vi "ReadNet_ONXX.vi"(8 "error in":errorcluster, 11 "ModelPath":path) -> (0 "error out":errorcluster, 3 "NET":refnum<class "NET.lvclass">)   [LabVIEW 2020, in "OpenLvVision_OpenCv.lvlib"]
doc: "Reads a network model ONNX."
uses:
  OpenLvVision_OpenCv.lvlib
  NET/NET.lvclass
  _LvHelpers/EdvrObject/TypeDef/Edvr.ctl
  _LvHelpers/EdvrObject/EdvrObject.lvclass
  Dlls/OlvOpenCvWrapper.dll
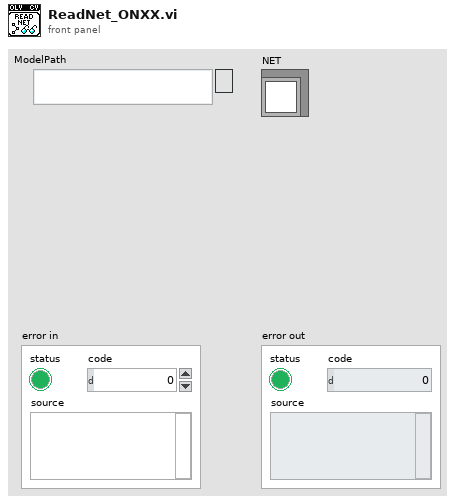
[diagram p1: front panel]
types:
  T1 = typedef "OpenLvVision_OpenCv.lvlib/EdvrObject.lvclass/Edvr.ctl" = refnum<data-value>
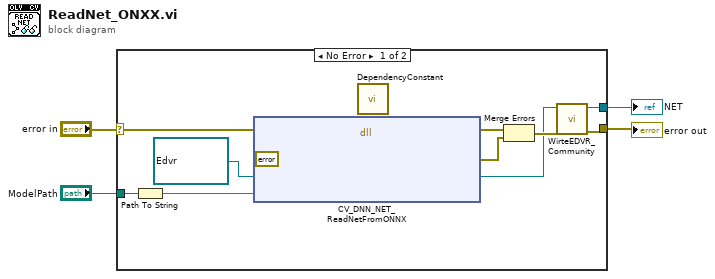
[diagram p0: block diagram]
diagram:
  n1 = case shown="No Error" "error in" {
    selector: "error in" -> [w12 w16]
    tunnel: [w10 w16] -> w3
    tunnel: [w8 _] -> w2
    tunnel: "ModelPath" -> [w7 _]
    frame No Error {
      n2 = Path To String(path=w7) -> (string=w6:string)
      n3 = dll-call lib="C:/Users/lukas/Downloads/OpenLvVision_OpenCv/SourceCode/LabView/OpenLvVision_OpenCv/Dlls/OlvOpenCvWrapper.dll" fn="CV_DNN_NET_ReadNetFromONNX"(error in=w12, "Error"=errorcluster {"status"=FALSE, "code"=0, "source"=""} ("error out"), "edvrRef"=T1 refnum ("Edvr"), "modelPath"=w6) -> (error out=w14:errorcluster, "Error"=w5:errorcluster, "edvrRef"=w9:T1)  [unwired: 4 in, 1 out]
      n4 = call "DependencyConstant.vi"() -> ()  [unwired: 12 in]
      n5 = Merge Errors(w14, w5) -> (w11:errorcluster)
      n6 = call "WirteEDVR_Community.vi"("error in"=w11, "Edvr"=w9) -> ("error out"=w10:errorcluster, "NET"=w8:refnum<class "NET.lvclass">)  [unwired: 8 in]
    }
    frame Error {
    }
  }
  "NET" <- w2
  "error out" <- w3
